vi "GLdrv_MEAS_OUTP_HEAD.vi"(0 "Connection ID":T1, 11 "error in (no error)":errorcluster) -> (4 "Connection ID Out":T1, 6 "Header out":string, 15 "error out":errorcluster)   [LabVIEW 2017, in "GL860_Driver.lvlib"]
doc: "リアルタイムデータをファイル化する際のデータヘッダを転送します\n　（ヘッダの内容は別紙参照）"
uses:
  GL860_Driver.lvlib
  ConnectionID.ctl
  GLdrv_RW.ctl
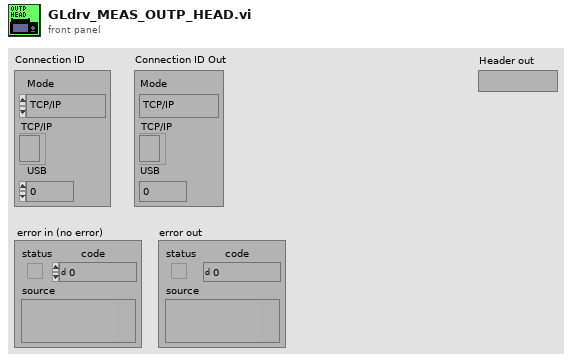
[diagram p1: front panel]
types:
  T1 = typedef "ConnectionID.ctl" = cluster{"Mode":enum16{"TCP/IP", "USB"}, "TCP/IP":refnum<k5>, "USB":i32}
  T2 = typedef "GLdrv_RW.ctl" = enum16{"Auto", "Read", "Write", "Buffer"}
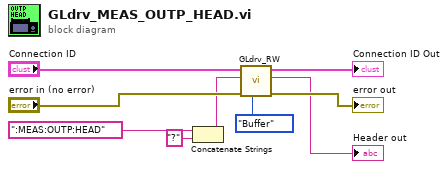
[diagram p0: block diagram]
diagram:
  n1 = Concatenate Strings(":MEAS:OUTP:HEAD" ("Command"), "?" ("string")) -> (w3:string)
  n2 = call "GLdrv_RW.vi"("Mode(read)"=GLdrv_RW."Buffer", "error in (no error)"="error in (no error)", "data in"=w3, "Connection ID"="Connection ID") -> ("error out"=→"error out":errorcluster, "data out"=→"Header out":string, "Connection ID Out"=→"Connection ID Out":T1)  [unwired: 3 in, 2 out]
